vi "test-transform2d.vi"(8 "error in (no error)":errorcluster) -> (0 "error out":errorcluster, 3 "All PASSED":bool)   [LabVIEW 2019]
uses:
  <vilib>/Rock Robotics/WPI/ThirdParty/JAS_Junk/TrajLib/Transform2d_Create_PosePose.vi
  <vilib>/Rock Robotics/WPI/ThirdParty/JAS_Junk/TrajLib/Pose2d_New.vi
  <vilib>/Rock Robotics/WPI/ThirdParty/JAS_Junk/TrajLib/Pose2d_TransformBy.vi
  <vilib>/Rock Robotics/WPI/ThirdParty/JAS_Junk/TrajLib/Translation2d_Equals.vi
  <vilib>/Rock Robotics/WPI/ThirdParty/JAS_Junk/TrajLib/Rotation2d_Equals.vi
  <vilib>/Rock Robotics/WPI/ThirdParty/JAS_Junk/TrajLib/Translation2d_UnaryMinus.vi
  <vilib>/Rock Robotics/WPI/ThirdParty/JAS_Junk/TrajLib/Rotation2d_UnaryMinus.vi
  <vilib>/Rock Robotics/WPI/ThirdParty/JAS_Junk/TrajLib/Translation2d_RotateBy.vi
  <vilib>/Rock Robotics/WPI/ThirdParty/JAS_Junk/TrajLib/Translation2d_Minus.vi
  <vilib>/Rock Robotics/WPI/ThirdParty/JAS_Junk/TrajLib/Rotation2d_Minus.vi
  <vilib>/Rock Robotics/WPI/ThirdParty/JAS_Junk/TrajLib/Translation2d_Plus.vi
  <vilib>/Rock Robotics/WPI/ThirdParty/JAS_Junk/TrajLib/Rotation2d_Plus.vi
  <vilib>/Rock Robotics/WPI/ThirdParty/JAS_Junk/TrajLib/Util_CalcDist.vi
  <vilib>/Rock Robotics/WPI/ThirdParty/JAS_Junk/TrajLib/Rotation2d_RotateBy.vi
  <vilib>/Rock Robotics/WPI/ThirdParty/JAS_Junk/TrajLib/Rotation2d_CreateXY.vi
  <vilib>/Rock Robotics/WPI/ThirdParty/JAS_Junk/TrajLib/Trajectory_Library.lvlib
panel:
  out "Test 2 Passed":bool
  out "T1 Passed":bool
  out "T5 - ANG = 43 Deg":dbl
  out "T5 - Y2 = 4.4":dbl
  out "T5 - X2= -3.33":dbl
  out "T5 - Y = 4.4":dbl
  out "T5 - X = -3.33":dbl
  # "Transform2D Test  --- NOT DONE"
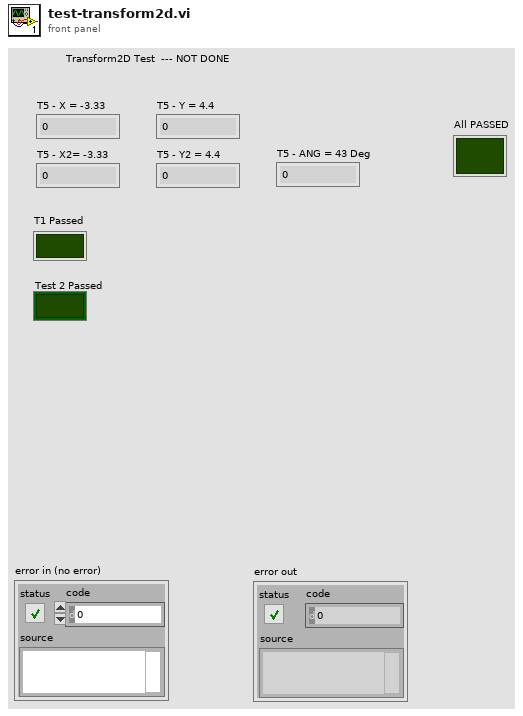
[diagram p1: front panel]
types:
  T1 = typedef "Trajectory_Library.lvlib/TRANSLATION2D.ctl" = cluster{"X":dbl, "Y":dbl}
  T2 = typedef "Trajectory_Library.lvlib/ROTATION2D.ctl" = cluster{"VALUE":dbl, "COS":dbl, "SIN":dbl}
  T3 = typedef "Trajectory_Library.lvlib/TRANSFORM2D.ctl" = cluster{"TRANSLATION":T1, "ROTATION":T2}
  T4 = typedef "Trajectory_Library.lvlib/POSE2D.ctl" = cluster{"TRANSLATION":T1, "ROTATION":T2}
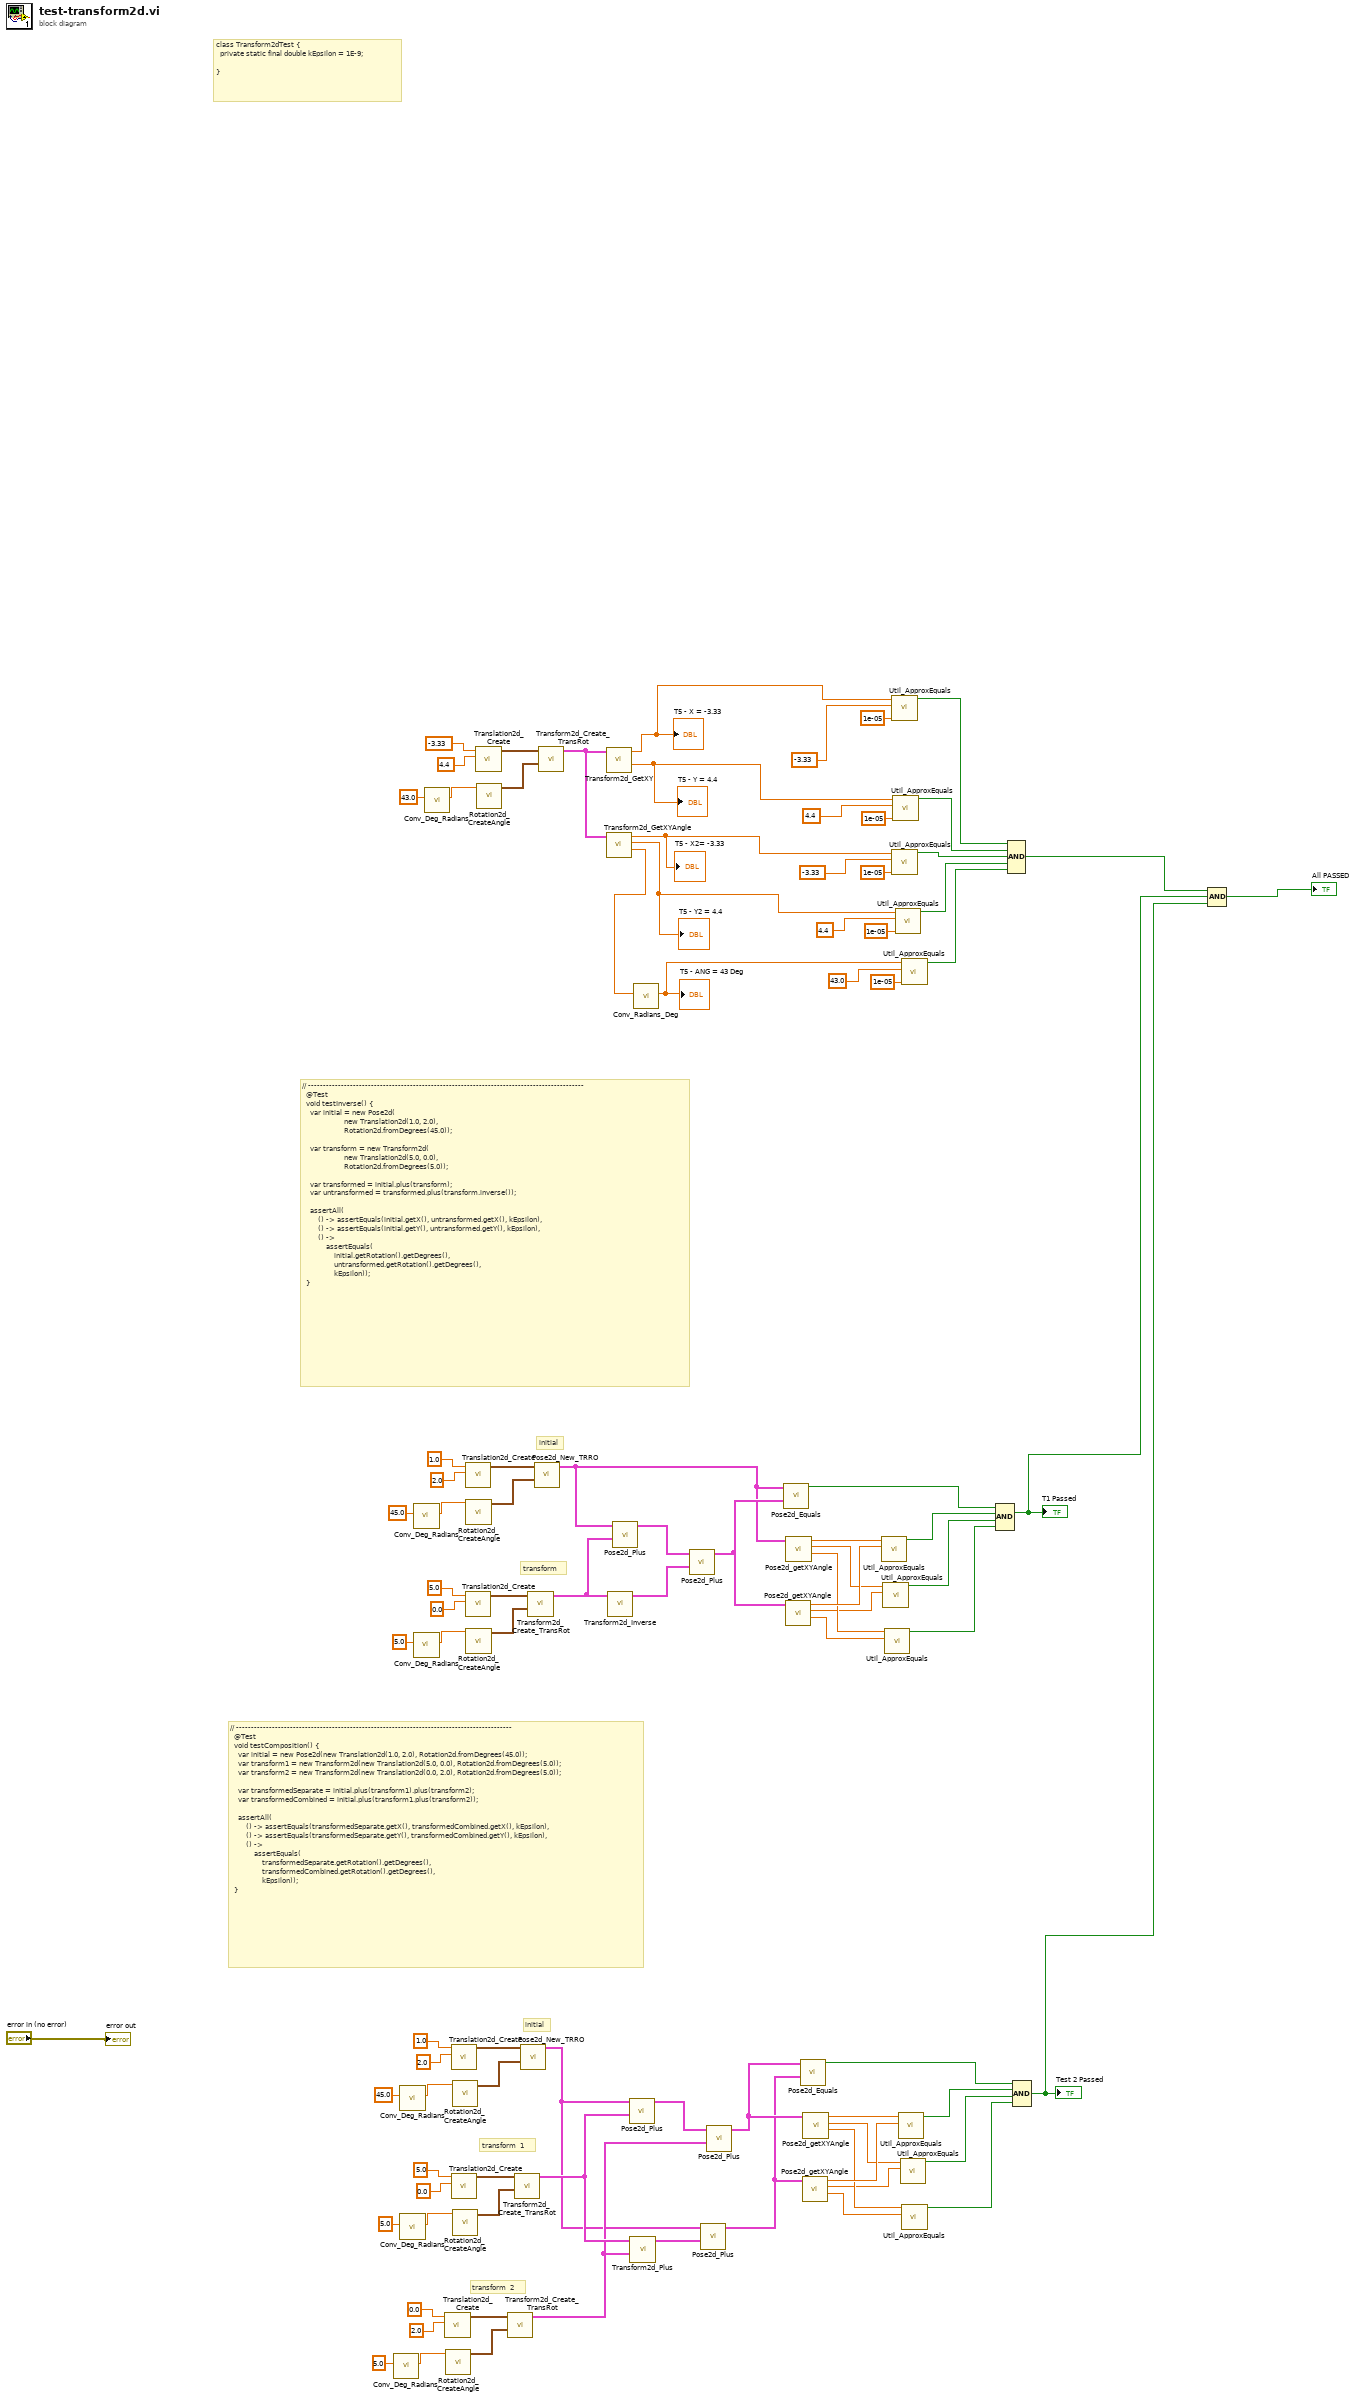
[diagram p0: block diagram]
diagram:
  # "transform  2"
  # "transform  1"
  # "initial"
  # "transform"
  # "initial"
  # "// --------------------------------------------------------------------------------------------\n  @Test\n  void testComposition() {\n    var initial = new Pose2d(new Translation2d(1.0, 2.0), Rotation2d.fromDegrees(45.0));\n    var transform1 = new Transform2d(new Translation2d(5.0, 0.0), Rotation2d.fromDegrees(5.0));\n    var transform2 = new Transform2d(new Translation2d(0.0, 2.0), Rotation2d.fromDegrees(5.0));\n\n    var transformedSeparate = initial.plus(transform1).plus(transform2);\n    var transformedCombined = initial.plus(transform1.plus(transform2));\n\n    assertAll(\n        () -> assertEquals(transformedSeparate.getX(), transformedCombined.getX(), kEpsilon),\n        () -> assertEquals(transformedSeparate.getY(), transformedCombined.getY(), kEpsilon),\n        () ->\n            assertEquals(\n                transformedSeparate.getRotation().getDegrees(),\n                transformedCombined.getRotation().getDegrees(),\n                kEpsilon));\n  }"
  # "// --------------------------------------------------------------------------------------------\n  @Test\n  void testInverse() {\n    var initial = new Pose2d(\n                     new Translation2d(1.0, 2.0), \n                     Rotation2d.fromDegrees(45.0));\n\n    var transform = new Transform2d(\n                     new Translation2d(5.0, 0.0), \n                     Rotation2d.fromDegrees(5.0));\n\n    var transformed = initial.plus(transform);\n    var untransformed = transformed.plus(transform.inverse());\n\n    assertAll(\n        () -> assertEquals(initial.getX(), untransformed.getX(), kEpsilon),\n        () -> assertEquals(initial.getY(), untransformed.getY(), kEpsilon),\n        () ->\n            assertEquals(\n                initial.getRotation().getDegrees(),\n                untransformed.getRotation().getDegrees(),\n                kEpsilon));\n  }"
  # "class Transform2dTest {\n  private static final double kEpsilon = 1E-9;\n\n}"
  n1 = call <vilib>:"Conv_Deg_Radians.vi"("Degress"=5.0) -> ("Radians"=w17:dbl)  [unwired: 10 in]
  n2 = call <vilib>:"Conv_Deg_Radians.vi"("Degress"=45.0) -> ("Radians"=w40:dbl)  [unwired: 10 in]
  n3 = call <vilib>:"Conv_Deg_Radians.vi"("Degress"=5.0) -> ("Radians"=w36:dbl)  [unwired: 10 in]
  n4 = call <vilib>:"Conv_Deg_Radians.vi"("Degress"=45.0) -> ("Radians"=w67:dbl)  [unwired: 10 in]
  n5 = call <vilib>:"Conv_Deg_Radians.vi"("Degress"=5.0) -> ("Radians"=w63:dbl)  [unwired: 10 in]
  n6 = call <vilib>:"Conv_Deg_Radians.vi"("Degress"=43.0) -> ("Radians"=w92:dbl)  [unwired: 10 in]
  n7 = call <vilib>:"Translation2d_Create.vi"("Y"=2.0, "X"=0.0) -> ("TRANSLATION"=w16:T1)  [unwired: 9 in]
  n8 = call <vilib>:"Rotation2d_CreateAngle.vi"("Angle"=w17) -> ("ROTATION"=w15:T2)  [unwired: 10 in]
  n9 = call <vilib>:"Translation2d_Create.vi"("Y"=2.0, "X"=1.0) -> ("TRANSLATION"=w33:T1)  [unwired: 9 in]
  n10 = call <vilib>:"Translation2d_Create.vi"("Y"=0.0, "X"=5.0) -> ("TRANSLATION"=w35:T1)  [unwired: 9 in]
  n11 = call <vilib>:"Rotation2d_CreateAngle.vi"("Angle"=w40) -> ("ROTATION"=w32:T2)  [unwired: 10 in]
  n12 = call <vilib>:"Rotation2d_CreateAngle.vi"("Angle"=w36) -> ("ROTATION"=w34:T2)  [unwired: 10 in]
  n13 = call <vilib>:"Translation2d_Create.vi"("Y"=2.0, "X"=1.0) -> ("TRANSLATION"=w60:T1)  [unwired: 9 in]
  n14 = call <vilib>:"Translation2d_Create.vi"("Y"=0.0, "X"=5.0) -> ("TRANSLATION"=w62:T1)  [unwired: 9 in]
  n15 = call <vilib>:"Rotation2d_CreateAngle.vi"("Angle"=w67) -> ("ROTATION"=w59:T2)  [unwired: 10 in]
  n16 = call <vilib>:"Rotation2d_CreateAngle.vi"("Angle"=w63) -> ("ROTATION"=w61:T2)  [unwired: 10 in]
  n17 = call <vilib>:"Translation2d_Create.vi"("Y"=4.4, "X"=-3.33) -> ("TRANSLATION"=w91:T1)  [unwired: 9 in]
  n18 = call <vilib>:"Rotation2d_CreateAngle.vi"("Angle"=w92) -> ("ROTATION"=w90:T2)  [unwired: 10 in]
  n19 = call <vilib>:"Transform2d_Create_TransRot.vi"("ROTATION"=w15, "TRANSLATION"=w16) -> ("TRANSFORM"=w13:T3)  [unwired: 9 in]
  n20 = call <vilib>:"Transform2d_Create_TransRot.vi"("ROTATION"=w34, "TRANSLATION"=w35) -> ("TRANSFORM"=w14:T3)  [unwired: 9 in]
  n21 = call <vilib>:"Pose2d_New_TRRO.vi"("ROTATION"=w32, "TRANSLATION"=w33) -> ("outPOSE"=w11:T4)  [unwired: 9 in]
  n22 = call <vilib>:"Transform2d_Create_TransRot.vi"("ROTATION"=w61, "TRANSLATION"=w62) -> ("TRANSFORM"=w57:T3)  [unwired: 9 in]
  n23 = call <vilib>:"Pose2d_New_TRRO.vi"("ROTATION"=w59, "TRANSLATION"=w60) -> ("outPOSE"=w54:T4)  [unwired: 9 in]
  n24 = call <vilib>:"Transform2d_Create_TransRot.vi"("ROTATION"=w90, "TRANSLATION"=w91) -> ("TRANSFORM"=w89:T3)  [unwired: 9 in]
  n25 = call <vilib>:"Transform2d_GetXY.vi"("inTRANSFORM"=w89) -> ("Y"=w79:dbl, "X"=w86:dbl)  [unwired: 9 in]
  "T5 - X = -3.33" <- w86
  "T5 - Y = 4.4" <- w79
  n26 = call <vilib>:"Transform2d_GetXYAngle.vi"("inTRANSFORM"=w89) -> ("Angle"=w88:dbl, "Y"=w75:dbl, "X"=w77:dbl)  [unwired: 8 in]
  "T5 - X2= -3.33" <- w77
  "T5 - Y2 = 4.4" <- w75
  n27 = call <vilib>:"Transform2d_Inverse.vi"("inTRANSFORM"=w57) -> ("TRANSFORM"=w56:T3)  [unwired: 10 in]
  n28 = call <vilib>:"Pose2d_Plus.vi"("other TRANSFORM"=w57, "in POSE"=w54) -> ("out POSE"=w58:T4)  [unwired: 9 in]
  n29 = call <vilib>:"Pose2d_Plus.vi"("other TRANSFORM"=w14, "in POSE"=w11) -> ("out POSE"=w31:T4)  [unwired: 9 in]
  n30 = call <vilib>:"Transform2d_Plus.vi"("otherTRANSFORM"=w13, "inTRANSFORM"=w14) -> ("TRANSFORM"=w12:T3)  [unwired: 9 in]
  n31 = call <vilib>:"Conv_Radians_Deg.vi"("Radians"=w88) -> ("Degrees"=w73:dbl)  [unwired: 10 in]
  "T5 - ANG = 43 Deg" <- w73
  n32 = call <vilib>:"Pose2d_Plus.vi"("other TRANSFORM"=w56, "in POSE"=w58) -> ("out POSE"=w55:T4)  [unwired: 9 in]
  n33 = call <vilib>:"Pose2d_Plus.vi"("other TRANSFORM"=w12, "in POSE"=w11) -> ("out POSE"=w9:T4)  [unwired: 9 in]
  n34 = call <vilib>:"Pose2d_Plus.vi"("other TRANSFORM"=w13, "in POSE"=w31) -> ("out POSE"=w10:T4)  [unwired: 9 in]
  n35 = call <vilib>:"Pose2d_Equals.vi"("other POSE"=w55, "in POSE"=w54) -> ("Equals"=w50:bool)  [unwired: 9 in]
  n36 = call <vilib>:"Pose2d_getXYAngle.vi"("in POSE"=w55) -> ("Angle"=w45:dbl, "Y"=w46:dbl, "X"=w52:dbl)  [unwired: 8 in]
  n37 = call <vilib>:"Pose2d_getXYAngle.vi"("in POSE"=w54) -> ("Angle"=w47:dbl, "Y"=w51:dbl, "X"=w53:dbl)  [unwired: 8 in]
  n38 = call <vilib>:"Pose2d_Equals.vi"("other POSE"=w9, "in POSE"=w10) -> ("Equals"=w27:bool)  [unwired: 9 in]
  n39 = call <vilib>:"Pose2d_getXYAngle.vi"("in POSE"=w9) -> ("Angle"=w22:dbl, "Y"=w23:dbl, "X"=w29:dbl)  [unwired: 8 in]
  n40 = call <vilib>:"Pose2d_getXYAngle.vi"("in POSE"=w10) -> ("Angle"=w24:dbl, "Y"=w28:dbl, "X"=w30:dbl)  [unwired: 8 in]
  n41 = call <vilib>:"Util_ApproxEquals.vi"("Value 2"=w52, "Value 1"=w53) -> ("ApproxEquals"=w49:bool)  [unwired: 9 in]
  n42 = call <vilib>:"Util_ApproxEquals.vi"("Value 2"=w46, "Value 1"=w51) -> ("ApproxEquals"=w48:bool)  [unwired: 9 in]
  n43 = call <vilib>:"Util_ApproxEquals.vi"("Value 2"=w45, "Value 1"=w47) -> ("ApproxEquals"=w44:bool)  [unwired: 9 in]
  n44 = call <vilib>:"Util_ApproxEquals.vi"("Tolerance"=1e-05, "Value 2"=-3.33 ("y"), "Value 1"=w86) -> ("ApproxEquals"=w6:bool)  [unwired: 8 in]
  n45 = call <vilib>:"Util_ApproxEquals.vi"("Tolerance"=1e-05, "Value 2"=-3.33 ("y"), "Value 1"=w77) -> ("ApproxEquals"=w3:bool)  [unwired: 8 in]
  n46 = call <vilib>:"Util_ApproxEquals.vi"("Tolerance"=1e-05, "Value 2"=4.4 ("y"), "Value 1"=w79) -> ("ApproxEquals"=w4:bool)  [unwired: 8 in]
  n47 = call <vilib>:"Util_ApproxEquals.vi"("Tolerance"=1e-05, "Value 2"=4.4 ("y"), "Value 1"=w75) -> ("ApproxEquals"=w2:bool)  [unwired: 8 in]
  n48 = call <vilib>:"Util_ApproxEquals.vi"("Value 2"=w29, "Value 1"=w30) -> ("ApproxEquals"=w26:bool)  [unwired: 9 in]
  n49 = call <vilib>:"Util_ApproxEquals.vi"("Value 2"=w23, "Value 1"=w28) -> ("ApproxEquals"=w25:bool)  [unwired: 9 in]
  n50 = call <vilib>:"Util_ApproxEquals.vi"("Tolerance"=1e-05, "Value 2"=43.0 ("y"), "Value 1"=w73) -> ("ApproxEquals"=w1:bool)  [unwired: 8 in]
  n51 = call <vilib>:"Util_ApproxEquals.vi"("Value 2"=w22, "Value 1"=w24) -> ("ApproxEquals"=w21:bool)  [unwired: 9 in]
  n52 = Compound Arithmetic op=AND(w50, w49, w48, w44) -> (w8:bool)
  "T1 Passed" <- w8
  n53 = Compound Arithmetic op=AND(w6, w4, w3, w2, w1) -> (w5:bool)
  n54 = Compound Arithmetic op=AND(w27, w26, w25, w21) -> (w7:bool)
  "Test 2 Passed" <- w7
  n55 = Compound Arithmetic op=AND(w5, w8, w7) -> (→"All PASSED":bool)
  "error out" <- "error in (no error)"
